vi "Test Konfiguracja API.vi"() -> ()   [LabVIEW 2017]
doc: "Konfiguracja API Tester."
uses:
  Konfiguracja.lvlib
panel:
  in  "Show Block Diagram":bool
  in  "Stop Module":bool
  in  "Start Module":bool
  in  "Hide Module Panel":bool
  in  "Show Module Panel":bool
  out "Status":string
  out "Module Running?":bool
  # "This VI tests the API for the Module."
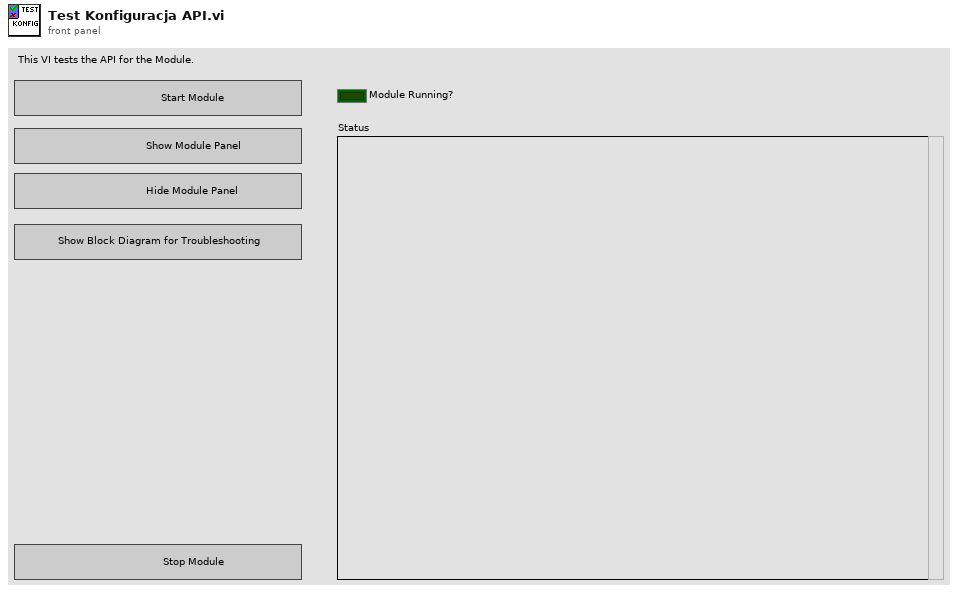
[diagram p1: front panel]
types:
  T1 = typedef "Konfiguracja.lvlib/Broadcast Events--cluster.ctl" = cluster{"Module Did Init":refnum<user-event>, "Status Updated":refnum<user-event>, "Error Reported":refnum<user-event>, "Module Did Stop":refnum<user-event>, "Update Module Execution Status":refnum<user-event>, "Subpanel VI Loaded":refnum<user-event>}
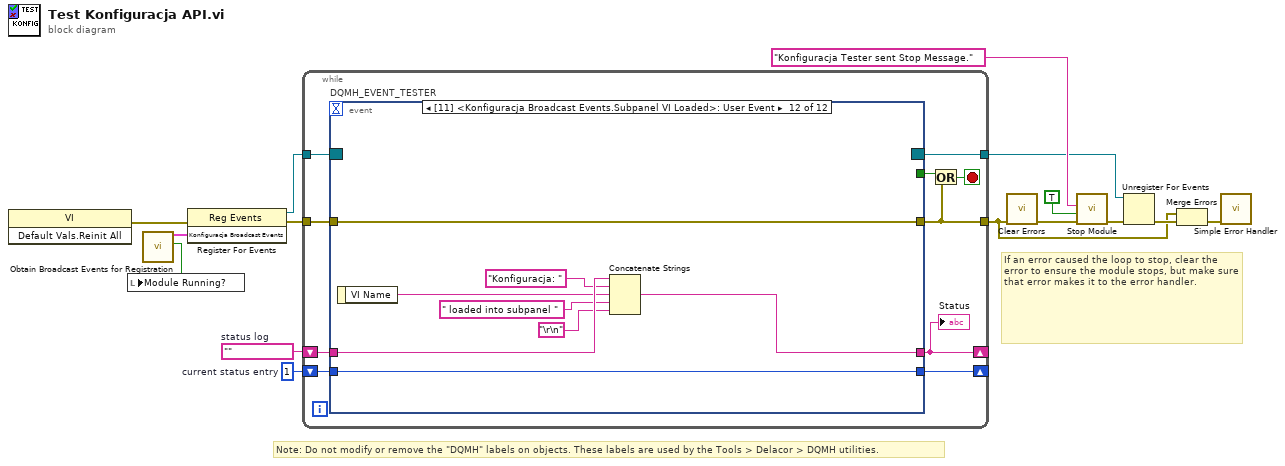
[diagram p0: block diagram]
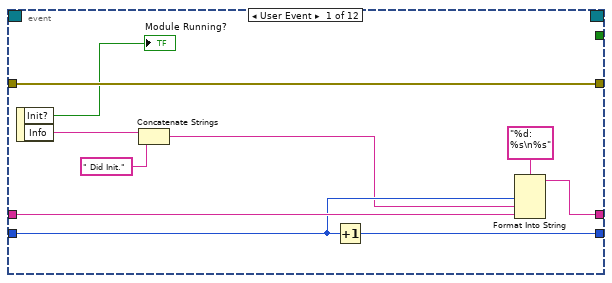
[diagram p2: hidden frame]
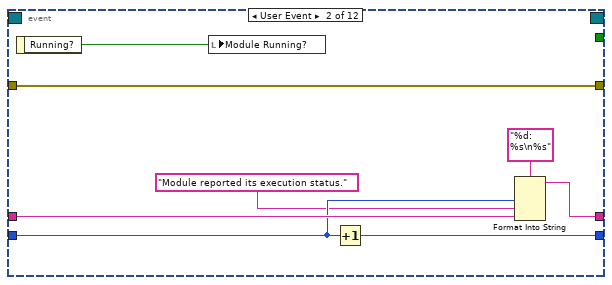
[diagram p3: hidden frame]
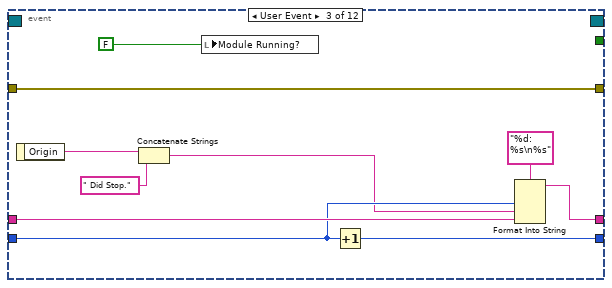
[diagram p4: hidden frame]
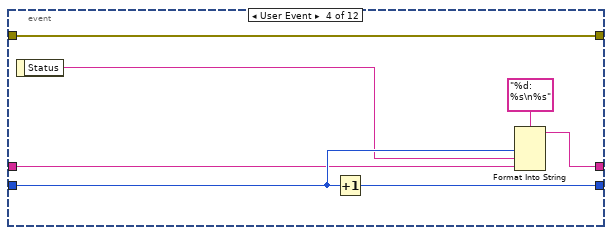
[diagram p5: hidden frame]
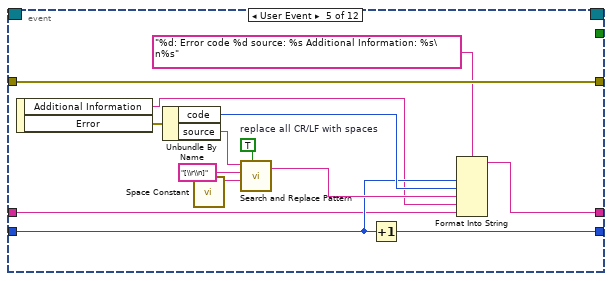
[diagram p6: hidden frame]
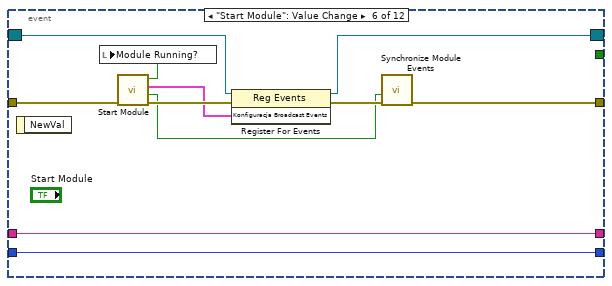
[diagram p7: hidden frame]
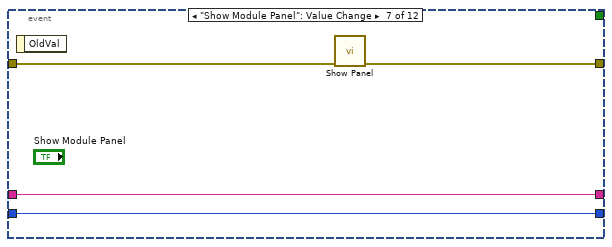
[diagram p8: hidden frame]
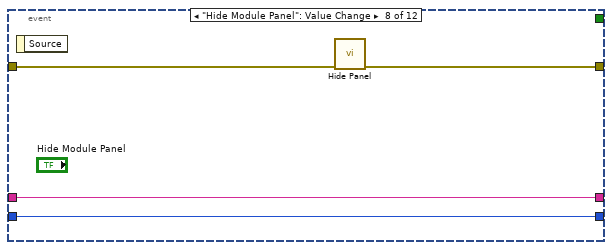
[diagram p9: hidden frame]
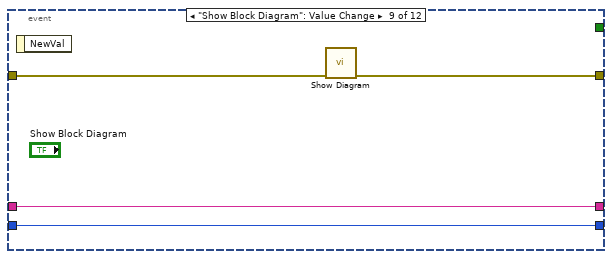
[diagram p10: hidden frame]
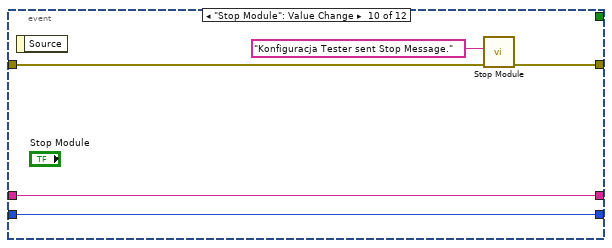
[diagram p11: hidden frame]
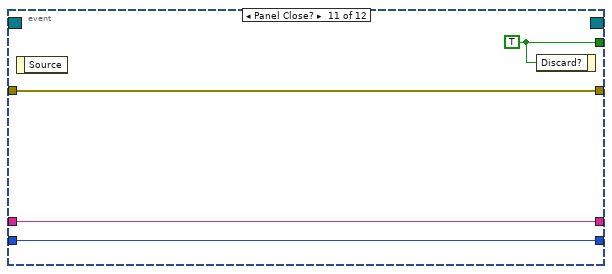
[diagram p12: hidden frame]
diagram:
  w11 = 1  # current status entry
  w12 = ""  # status log
  # "If an error caused the loop to stop, clear the error to ensure the module stops, but make sure that error makes it to the error handler."
  # "Note: Do not modify or remove the \"DQMH\" labels on objects. These labels are used by the Tools > Delacor > DQMH utilities."
  n1 = invoke class="VI" method="Default Vals.Reinit All"() -> (error out=w10:errorcluster)  [unwired: 3 in, 2 out]
  n2 = call "Obtain Broadcast Events for Registration.vi"() -> ("Already running?"=w1:bool, "Konfiguracja Broadcast Events"=w8:T1)  [unwired: 9 in, 1 out]
  n3 = local write "Module Running?"(w1) -> ()
  n4 = register-events(error in=w10, w8) -> (reference out=w7:refnum<event-registration>, error out=w9:errorcluster)  [unwired: 1 in]
  n5 = while {
    tunnel: w7 -> [w25]
    tunnel: [w16] -> w2
    shift-right: [w20] -> _
    shift-left: w12 -> [w22]
    shift-right: [w21] -> _
    shift-left: w11 -> [w23]
    tunnel: w9 -> [w18]
    tunnel: [w17] -> w6
    stop <- w19 stop-if-true
    n6 = event "DQMH_EVENT_TESTER" shown="[11] <Konfiguracja Broadcast Events.Subpanel VI Loaded>: User Event" {
      selector: w25 -> [_ _ _ _ _ w79 _ _ _ _ _ _]
      dyn-events: [_ _ _ _ _ w78 _ _ _ _ _ _] -> w17
      timeout: _ -> [_ _ _ _ _ _ _ _ _ _ _ _]
      tunnel: [_ _ _ _ _ _ _ _ _ _ w106 _] -> w24
      tunnel: [w35 w37 w44 w54 w74 w77 w89 w93 w94 w100 w103 w114] -> w16
      tunnel: w23 -> [w31 w41 w51 w57 w64 w82 w87 w91 w95 w101 w104 w112]
      tunnel: w22 -> [w32 w42 w52 w56 w62 w83 w88 w92 w96 w102 w105 w113]
      tunnel: [w29 w39 w49 w58 w65 w83 w88 w92 w96 w102 w105 w111] -> w20
      tunnel: [w30 w40 w50 w60 w63 w82 w87 w91 w95 w101 w104 w112] -> w21
      tunnel: w18 -> [w35 w37 w44 w54 w74 w76 w86 w90 w97 w98 w103 w114]
      event User Event {
        n7 = event-data() -> ("Init?"=→"Module Running?":bool, "Info"=w28:string)  [unwired: 1 in]
        n8 = Concatenate Strings(w28, " Did Init.") -> (w27:string)
        n9 = Increment(x=w31) -> (x+1=w30:i32)
        n10 = Format Into String(format string="%d: %s\n%s", w31, w27, w32) -> (resulting string=w29:string)  [unwired: 2 in, 1 out]
      }
      event User Event {
        n11 = event-data() -> ("Running?"=w36:bool)  [unwired: 1 in]
        n12 = local write "Module Running?"(w36) -> ()
        n13 = Increment(x=w41) -> (x+1=w40:i32)
        n14 = Format Into String(format string="%d: %s\n%s", w41, "Module reported its execution status.", w42) -> (resulting string=w39:string)  [unwired: 2 in, 1 out]
      }
      event User Event {
        n15 = event-data() -> ("Origin"=w48:string)  [unwired: 1 in]
        n16 = Concatenate Strings(w48, " Did Stop.") -> (w47:string)
        n17 = local write "Module Running?"(FALSE ("Module Did Init?")) -> ()
        n18 = Increment(x=w51) -> (x+1=w50:i32)
        n19 = Format Into String(format string="%d: %s\n%s", w51, w47, w52) -> (resulting string=w49:string)  [unwired: 2 in, 1 out]
      }
      event User Event {
        n20 = event-data() -> ("Status"=w55:string)  [unwired: 1 in]
        n21 = Increment(x=w57) -> (x+1=w60:i32)
        n22 = Format Into String(format string="%d: %s\n%s", w57, w55, w56) -> (resulting string=w58:string)  [unwired: 2 in, 1 out]
      }
      event User Event {
        w70 = TRUE  # replace all CR/LF with spaces
        n23 = event-data() -> ("Additional Information"=w61:string, "Error"=w66:errorcluster)  [unwired: 1 in]
        n24 = Unbundle By Name(w66) -> ("code"=w67:i32, "source"=w68:string)
        n25 = call <vilib>:"Space Constant.vi"() -> ("String"=w71:string)
        n26 = call <vilib>:"Search and Replace Pattern.vi"("string"=w68, "regular expression (\"\")"="[\\r\\n]" ("regular expression (\"\")"), "replace string (\"\")"=w71, "replace all? (F)"=w70) -> ("result string"=w69:string)  [unwired: 1 in, 1 out]
        n27 = Increment(x=w64) -> (x+1=w63:i32)
        n28 = Format Into String(format string="%d: Error code %d source: %s Additional Information: %s\n%s", w64, w67, w69, w61, w62) -> (resulting string=w65:string)  [unwired: 2 in, 1 out]
      }
      event "Start Module": Value Change {
        n29 = event-data() -> ()  [unwired: 1 in, 1 out]
        n30 = call "Start Module.vi"("error in (no error)"=w76) -> ("error out"=w84:errorcluster, "Wait for Event Sync?"=w81:bool, "Konfiguracja Broadcast Events"=w80:T1, "Module Was Already Running?"=w75:bool)  [unwired: 7 in]
        n31 = local write "Module Running?"(w75) -> ()
        n32 = register-events(reference=w79, error in=w84, w80) -> (reference out=w78:refnum<event-registration>, error out=w85:errorcluster)
        n33 = call "Synchronize Module Events.vi"("error in (no error)"=w85, "Wait for Event Sync?"=w81) -> ("error out"=w77:errorcluster)  [unwired: 9 in]
      }
      event "Show Module Panel": Value Change {
        n34 = event-data() -> ()  [unwired: 1 in, 1 out]
        n35 = call "Show Panel.vi"("error in (no error)"=w86) -> ("error out"=w89:errorcluster)  [unwired: 10 in]
      }
      event "Hide Module Panel": Value Change {
        n36 = event-data() -> ()  [unwired: 1 in, 1 out]
        n37 = call "Hide Panel.vi"("error in (no error)"=w90) -> ("error out"=w93:errorcluster)  [unwired: 10 in]
      }
      event "Show Block Diagram": Value Change {
        n38 = event-data() -> ()  [unwired: 1 in, 1 out]
        n39 = call "Show Diagram.vi"("error in (no error)"=w97) -> ("error out"=w94:errorcluster)  [unwired: 10 in]
      }
      event "Stop Module": Value Change {
        n40 = event-data() -> ()  [unwired: 1 in, 1 out]
        n41 = call "Stop Module.vi"("error in (no error)"=w98, "Origin"="Konfiguracja Tester sent Stop Message.") -> ("error out"=w100:errorcluster)  [unwired: 9 in]
      }
      event Panel Close? {
        w106 = TRUE ("Discard?")
        n42 = event-data() -> ()  [unwired: 1 in, 1 out]
        n43 = event-data("Discard?"=w106) -> ()  [unwired: 1 in, 1 out]
      }
      event User Event {
        n44 = event-data() -> ("VI Name"=w109:string)  [unwired: 1 in]
        n45 = Concatenate Strings(w113, "Konfiguracja: ", w109, " loaded into subpanel ", "\r\n") -> (w111:string)
      }
    }
    "Status" <- w20
    n46 = Or(x=w24, y=w16) -> (x .or. y?=w19:bool)
  }
  n47 = call <vilib>:"Clear Errors.vi"("error in (no error)"=w2) -> ("error out"=w4:errorcluster)  [unwired: 5 in, 1 out]
  n48 = call "Stop Module.vi"("error in (no error)"=w4, "Wait for Module to Stop? (F)"=TRUE ("Wait for Module to stop?"), "Origin"="Konfiguracja Tester sent Stop Message.") -> ("error out"=w14:errorcluster)  [unwired: 8 in]
  n49 = Unregister For Events(event registration refnum=w6, error in=w14) -> (error out=w15:errorcluster)
  n50 = Merge Errors(w2, w15) -> (w3:errorcluster)
  n51 = call <vilib>:"Simple Error Handler.vi"("error in (no error)"=w3) -> ()  [unwired: 4 in, 5 out]
